vi "Read Thread Queue.vi"(8 "error in (no error)":errorcluster, 11 "Thread in":refnum<class "Thread.lvclass">) -> (0 "error out":errorcluster, 1 "timed out?":bool, 2 "Message":refnum<class "Message.lvclass">, 3 "Thread out":refnum<class "Thread.lvclass">)   [LabVIEW 2019, in "Architecture.lvlib" / "Thread.lvclass"]
uses:
  Thread.lvclass
  Message/Message.lvclass
  Thread.lvclass/Thread.ctl
  Queue/Queue.lvclass
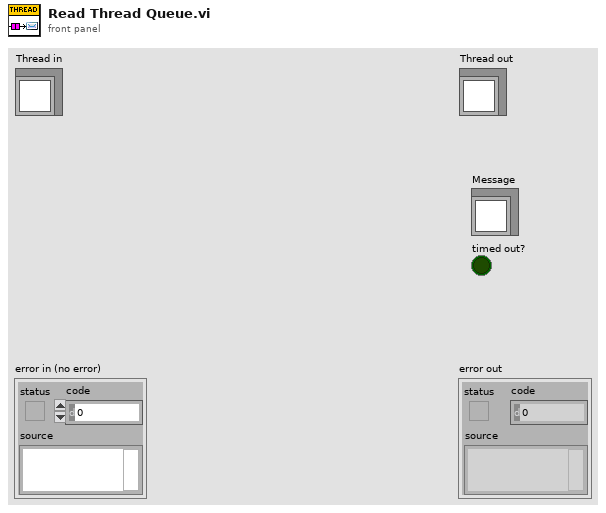
[diagram p1: front panel]
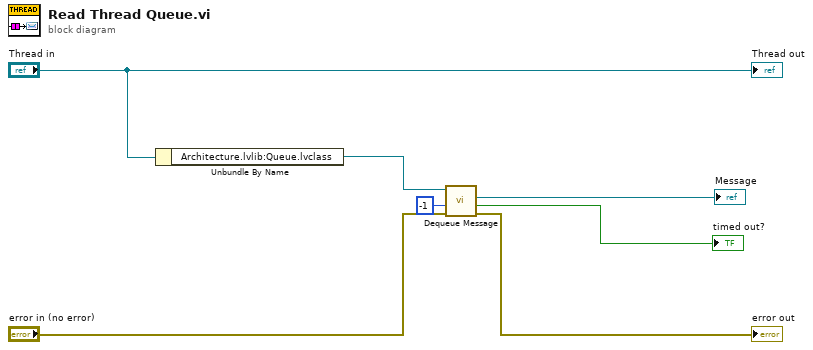
[diagram p0: block diagram]
diagram:
  n1 = Unbundle By Name("Thread in") -> ("Architecture.lvlib:Queue.lvclass"=w7:refnum<class "Queue.lvclass">)
  n2 = call "Dequeue Message.vi"("error in (no error)"="error in (no error)", "timeout in ms (-1)"=-1, "Queue in"=w7) -> ("error out"=→"error out":errorcluster, "timed out?"=→"timed out?":bool, "Message"=→"Message":refnum<class "Message.lvclass">)  [unwired: 5 in, 1 out]
  "Thread out" <- "Thread in"
